vi "Read Last Series Index.vi"(11 "Result in":refnum<class "Result.lvclass">) -> (2 "Series Index":i32, 3 "Result out":refnum<class "Result.lvclass">)   [LabVIEW 2018, in "InfluxDB Client.lvlib" / "Result.lvclass"]
uses:
  Result.lvclass
  Result.lvclass/Result.ctl
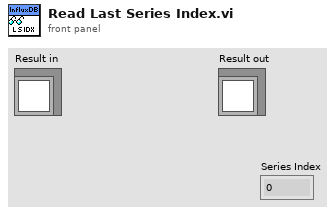
[diagram p1: front panel]
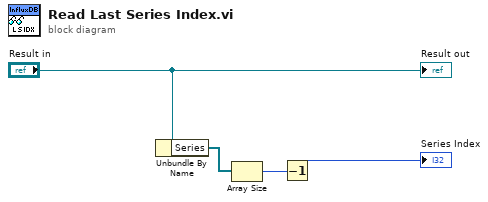
[diagram p0: block diagram]
diagram:
  n1 = Unbundle By Name("Result in") -> ("Series"=w3:refnum<class "Series.lvclass">[])
  n2 = Array Size(array=w3) -> (size(s)=w2:i32)
  n3 = Decrement(x=w2) -> (x-1=→"Series Index":i32)
  "Result out" <- "Result in"
